vi "Set VI Object Save Setting.vi"(8 "error in (no error)":errorcluster, 10 "Remove compiled code":bool, 11 "SDIST in":refnum<class "NI_AB_API_DSDIST.lvclass">) -> (0 "error out":errorcluster, 3 "SDIST out":refnum<class "NI_AB_API_DSDIST.lvclass">)   [LabVIEW 2020, in "NI_AB_API_DSDIST.lvclass"]
uses:
  <vilib>/AppBuilder/AB_API/DSDIST/NI_AB_API_DSDIST.lvclass
  <vilib>/AppBuilder/AB_API/SDIST/NI_AB_API_SDIST.lvclass
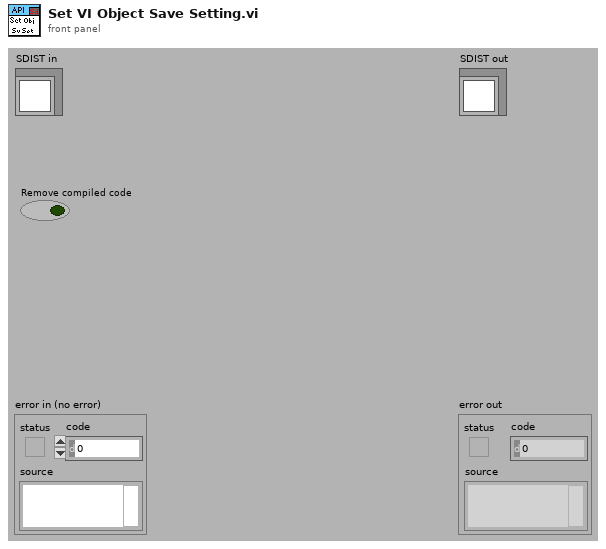
[diagram p1: front panel]
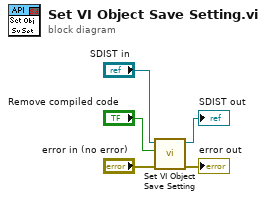
[diagram p0: block diagram]
diagram:
  n1 = call-parent "Set VI Object Save Setting.vi"("error in (no error)"="error in (no error)", "Remove compiled code"="Remove compiled code", "SDIST in"="SDIST in") -> ("error out"=→"error out":errorcluster, "SDIST out"=→"SDIST out":refnum<class "NI_AB_API_DSDIST.lvclass">)  [unwired: 7 in]
